vi "Write connection info.vi"(8 "error in (no error)":errorcluster, 10 "connection info":T1, 11 "AudioGeneration in":refnum<class "AudioGeneration.lvclass">) -> (0 "error out":errorcluster, 3 "AudioGeneration out":refnum<class "AudioGeneration.lvclass">)   [LabVIEW 2021, in "AudioGeneration.lvclass"]
uses:
  AudioGeneration.lvclass
  <vilib>/NI/STM/TCP/TCP Connection Info.ctl
  <vilib>/NI/STM/SubVIs/MetaDataElement.ctl
  AudioGeneration.lvclass/AudioGeneration.ctl
  <vilib>/NI/STM/NI STM.lvlib
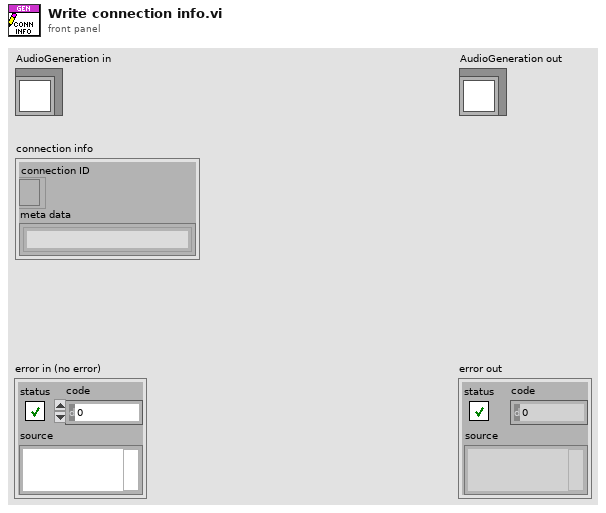
[diagram p1: front panel]
types:
  T1 = typedef "NI STM.lvlib/TCP Connection Info.ctl" = cluster{"connection ID":refnum<k5>, "meta data":T2[]}
  T2 = typedef "NI STM.lvlib/MetaDataElement.ctl" = string
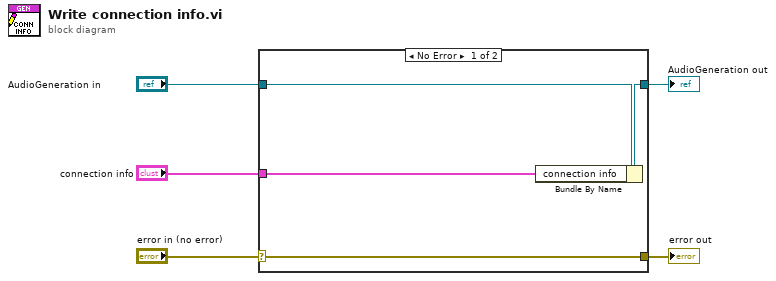
[diagram p0: block diagram]
diagram:
  n1 = case shown="No Error" "error in (no error)" {
    selector: "error in (no error)" -> [w9 w10]
    tunnel: [w9 w10] -> w4
    tunnel: [w7 w11] -> w2
    tunnel: "AudioGeneration in" -> [w8 w11]
    tunnel: "connection info" -> [w6 _]
    frame No Error {
      n2 = Bundle By Name(cluster=w8, "connection info"=w6) -> (w7:refnum<class "AudioGeneration.lvclass">)
    }
    frame Error {
    }
  }
  "error out" <- w4
  "AudioGeneration out" <- w2
